vi "Gestione_Inverter_VACON.vi"(6 "Inverter":refnum<vi>, 7 "Stato rpm":refnum<vi>, 8 "Test settings":refnum<vi>, 9 "RS485":refnum<vi>, 11 "name":string="VACON") -> ()   [LabVIEW 2019]
uses:
  Letture inverter.ctl
  Parametri inverter.ctl
  <vilib>/Modbus/subvis/Modbus API/Modbus API.lvclass/Modbus API.ctl
  <vilib>/Modbus/subvis/Transmission Data Unit (ADU)/Transmission Data Unit/Transmission Data Unit.lvclass/Transmission Data Unit.ctl
  <vilib>/Modbus/master/Data Access/Unit ID/Set Unit ID Property.vi
  <vilib>/Modbus/subvis/Transmission Data Unit (ADU)/Transmission Data Unit/Data Access/Unit ID/Write Unit ID.vi
  <vilib>/Modbus/subvis/Modbus API/Read Transmission Data Unit.vi
  <vilib>/Modbus/subvis/Modbus API/Write Transmission Data Unit.vi
  <vilib>/Modbus/master/Modbus Master.lvclass
  C:/Program Files (x86)/National Instruments/LabVIEW 2019/vi.lib/Modbus/subvis/Modbus API/Modbus API.lvclass
  <vilib>/Utility/file.llb/Read From Spreadsheet File (string).vi
  <vilib>/Modbus/master/Create Master Instance (Serial).vi
  STATUS VACON.vi
  <vilib>/Modbus/subvis/Transmission Data Unit (ADU)/Transmission Data Unit/Transmission Data Unit.lvclass
  Set inverter.ctl
panel:
  out "Cluster":T1
  out "senso rot":bool
  out "Boolean array":bool[](array[boolean])
  out "STATUS WORD":u16
  out "fREQ MAX":dbl
  in  "SET INVERTER":bool
  in  "Test settings 2":T2 caption="PARAMETRI INVERTER"
  in  "Scelta inverter":T3(radio)=enum."INVERTER 1 \n[7,5kW]"
  out "id":u8
  in  "stop":bool
  out "Numeric":i32
  out "status":string
  out "output cluster":T4
  out "error out":errorcluster
  # "Caratteristiche motore"
  # "Limiti massimi"
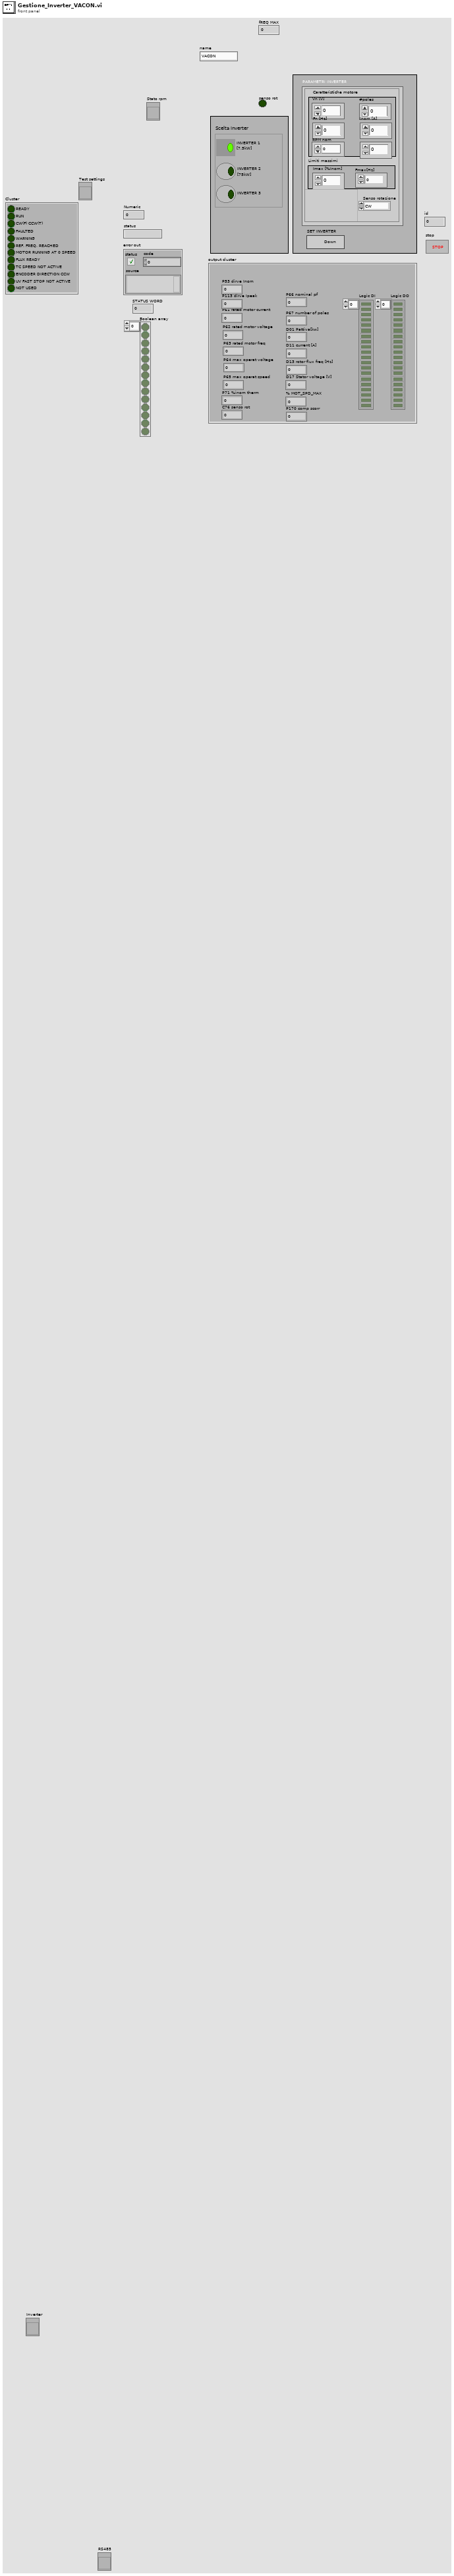
[diagram p1: front panel]
types:
  T1 = cluster{"READY":bool, "RUN":bool, "CW(F) CCW(T)":bool, "FAULTED":bool, "WARNING":bool, "REF. FREQ. REACHED":bool, "MOTOR RUNNING AT 0 SPEED":bool, "FLUX READY":bool, "TC SPEED NOT ACTIVE":bool, "ENCODER DIRECTION CCW":bool, "UV FAST STOP NOT ACTIVE":bool, "NOT USED":bool}
  T2 = typedef "Parametri inverter.ctl" = cluster{"Vn [V]":dbl, "Fn [Hz]":dbl, "CosFi":dbl, "Imax [%Inom]":dbl, "#poles":dbl, "Inom [A]":dbl, "Senso rotazione":enum16{"CW", "CCW"}, "RPM nom":dbl, "Fmax[Hz]":dbl}
  T3 = enum32{"No Selection", "INVERTER 1 \n[7,5kW]", "INVERTER 2 \n[75kW]", "INVERTER 3"}
  T4 = typedef "Letture inverter.ctl" = cluster{"P61 rated motor current":dbl, "P62 rated motor voltage":dbl, "P63 rated motor freq":dbl, "P64 max operat voltage":dbl, "P65 max operat speed":dbl, "P66 nominal pf":dbl, "P67 number of poles":dbl, "D01 Pattiva[kw]":dbl, "D11 current [A]":dbl, "D13 rotor flux freq [Hz]":dbl, "D17 Stator voltage [V]":dbl, "% MOT_SPD_MAX":dbl, "Logic DI":bool[], "Logic DO":bool[], "P71 %inom therm":dbl, "P53 dirve Inom":dbl, "P113 dirve Ipeak":dbl, "C76 senso rot":dbl, "P170 comp scorr":dbl}
  T5 = typedef "Set inverter.ctl" = cluster{"F [Hz]":dbl}
  T6 = cluster{"Boolean array[0]":bool, "Boolean array[1]":bool, "Boolean array[2]":bool, "Boolean array[3]":bool, "Boolean array[4]":bool, "Boolean array[5]":bool, "Boolean array[6]":bool, "Boolean array[7]":bool, "Boolean array[8]":bool, "Boolean array[9]":bool, "Boolean array[10]":bool, "Boolean array[11]":bool}
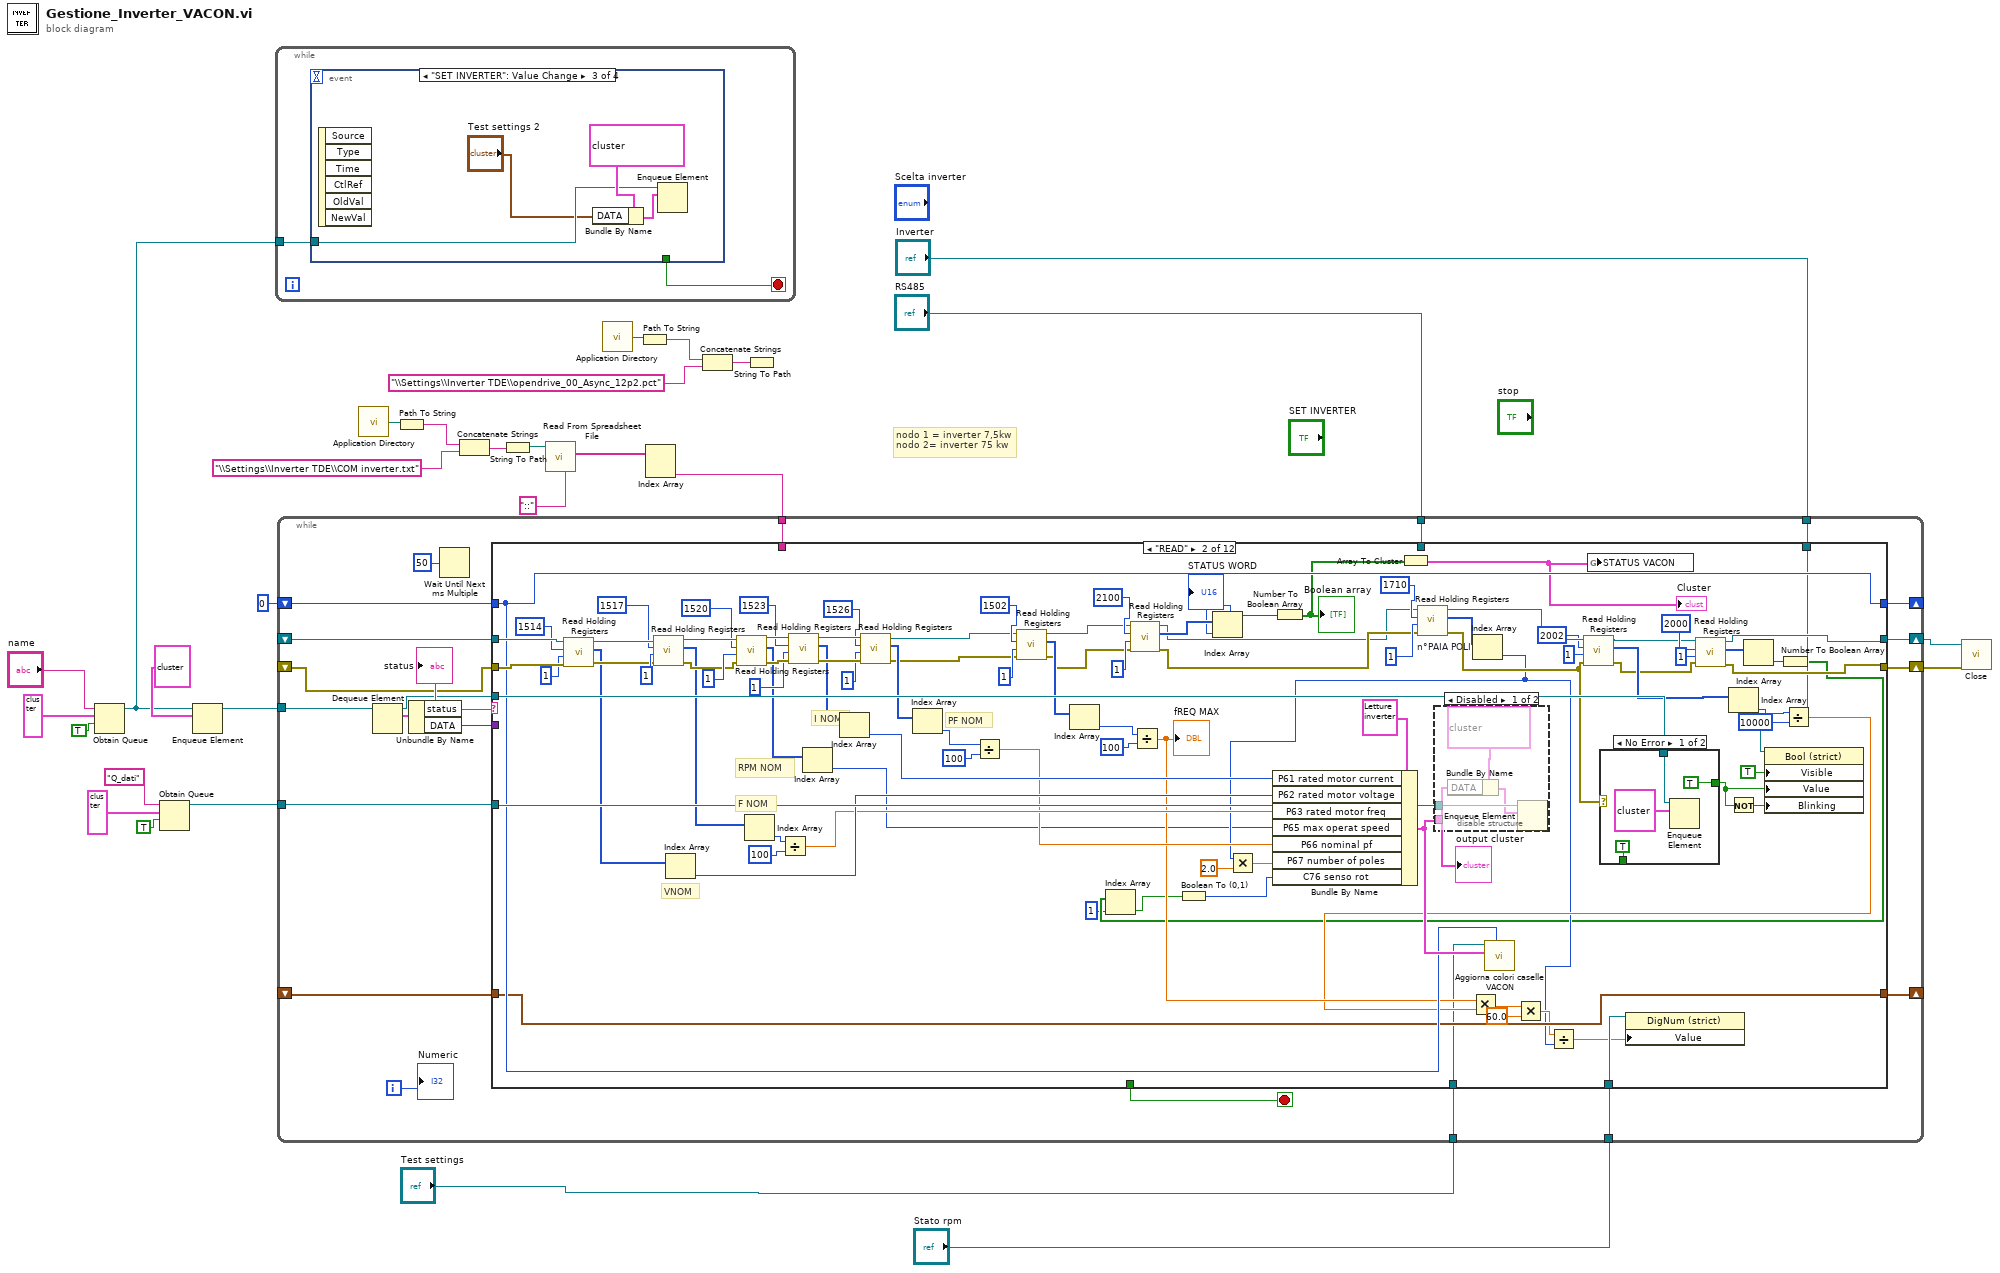
[diagram p0: block diagram]
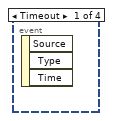
[diagram p2: hidden frame]
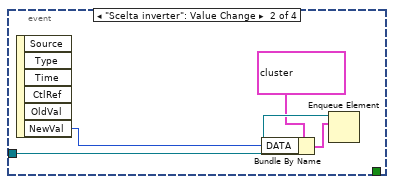
[diagram p3: hidden frame]
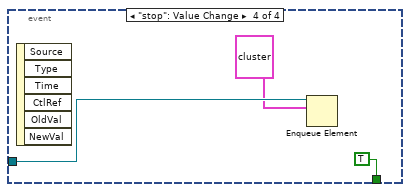
[diagram p4: hidden frame]
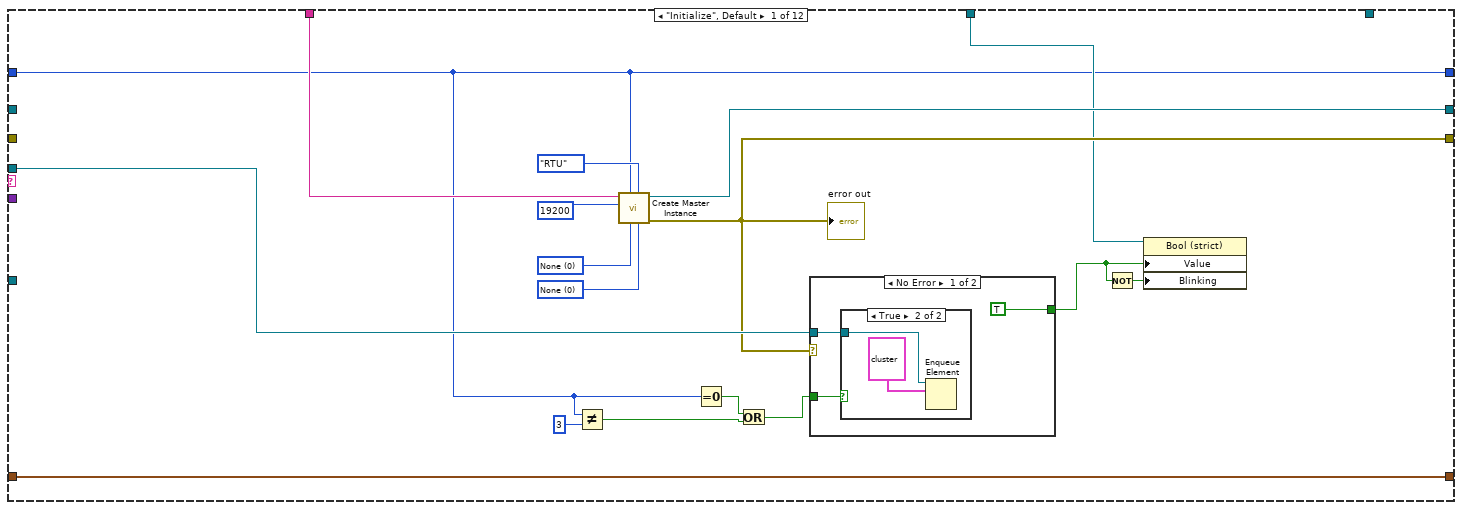
[diagram p5: hidden frame]
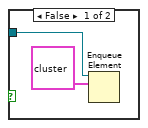
[diagram p6: hidden frame]
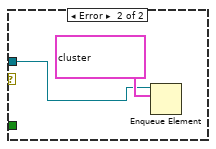
[diagram p7: hidden frame]
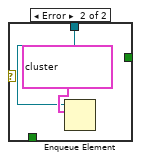
[diagram p9: hidden frame]
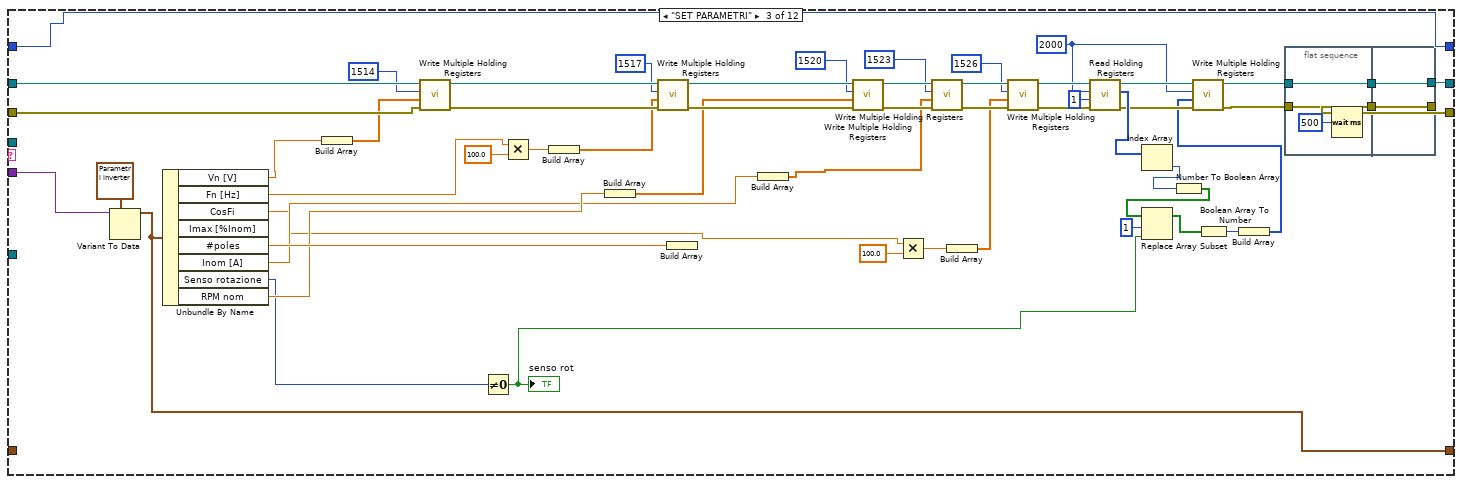
[diagram p10: hidden frame]
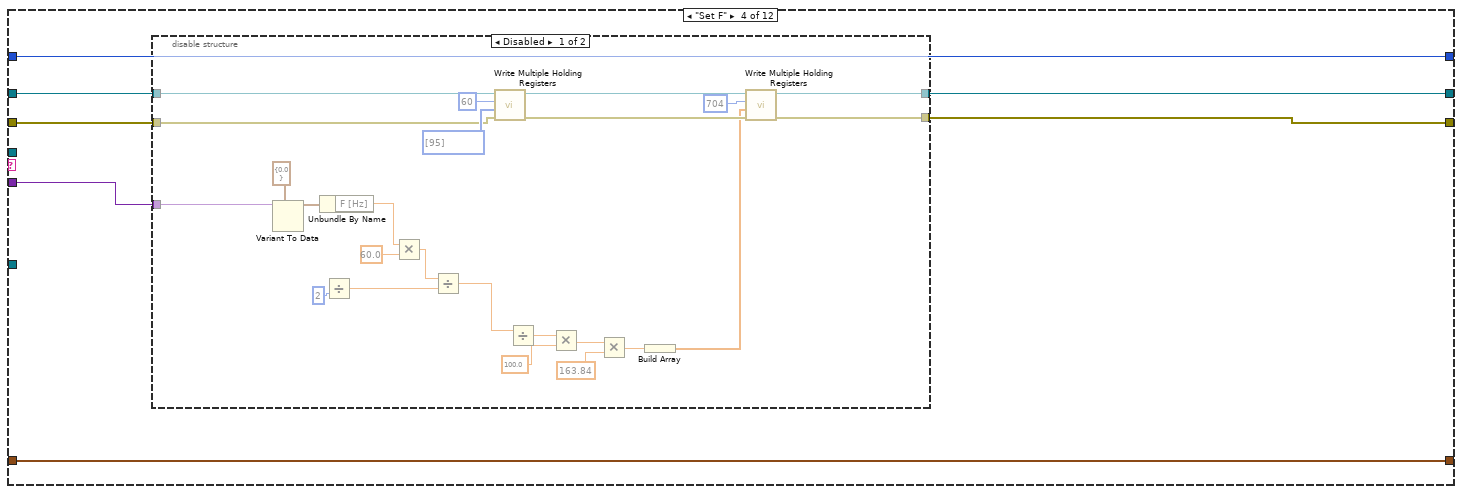
[diagram p11: hidden frame]
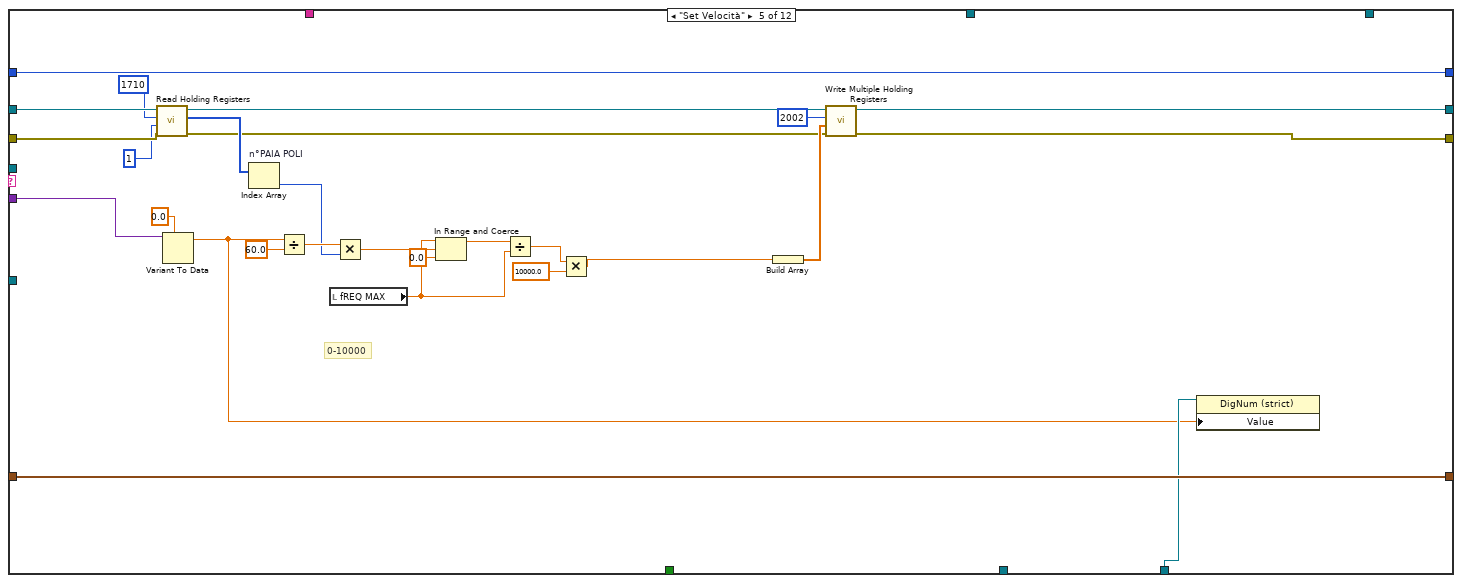
[diagram p13: hidden frame]
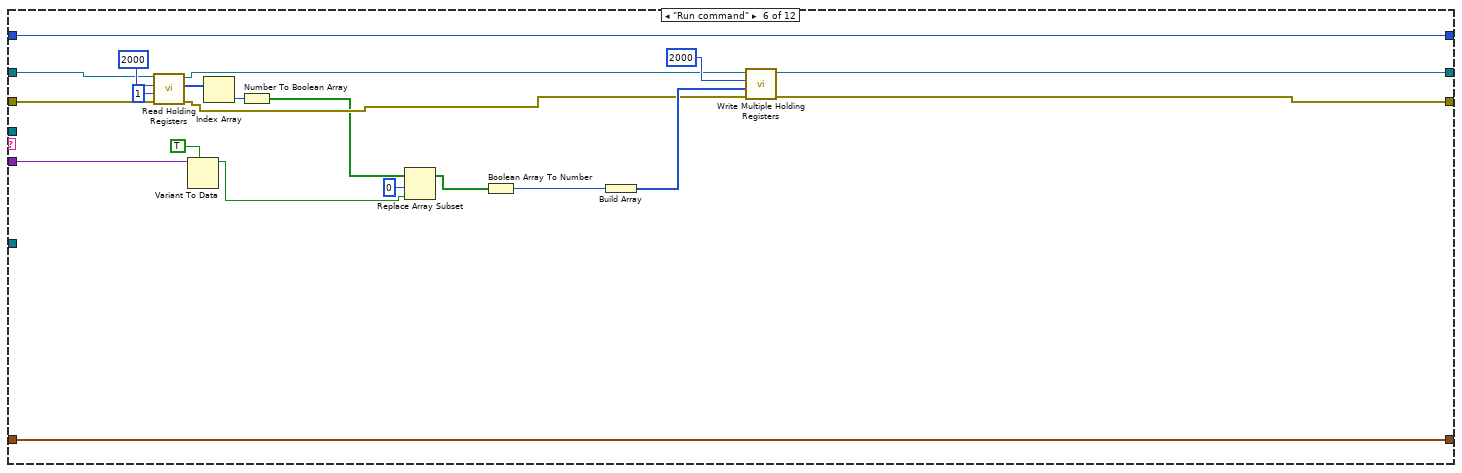
[diagram p14: hidden frame]
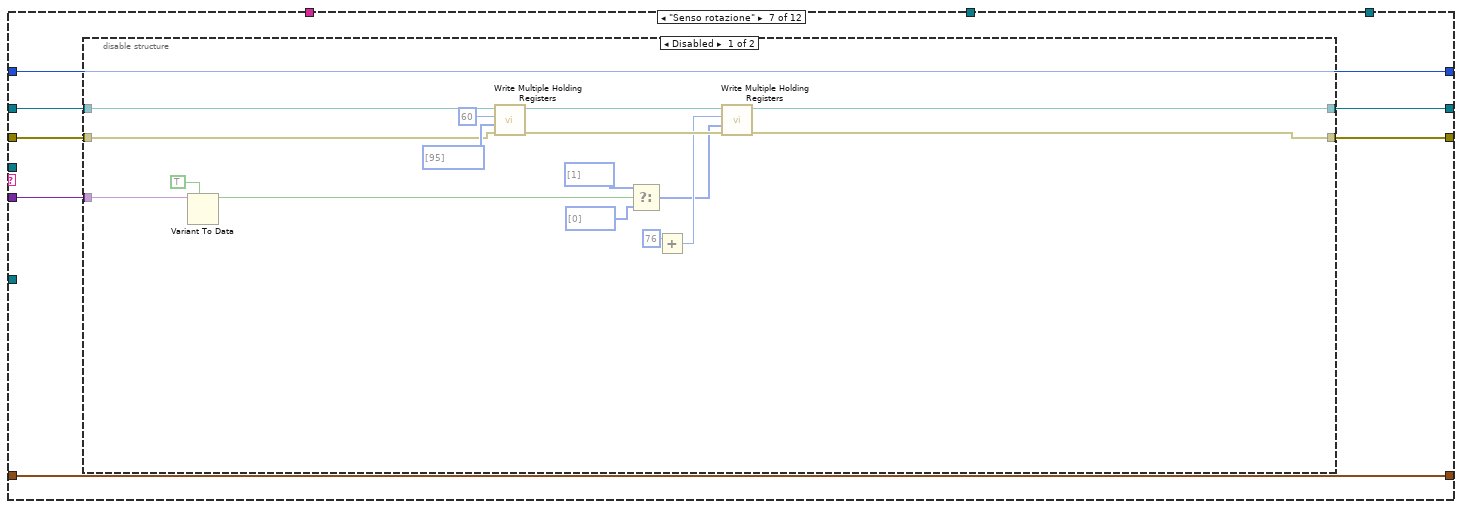
[diagram p15: hidden frame]
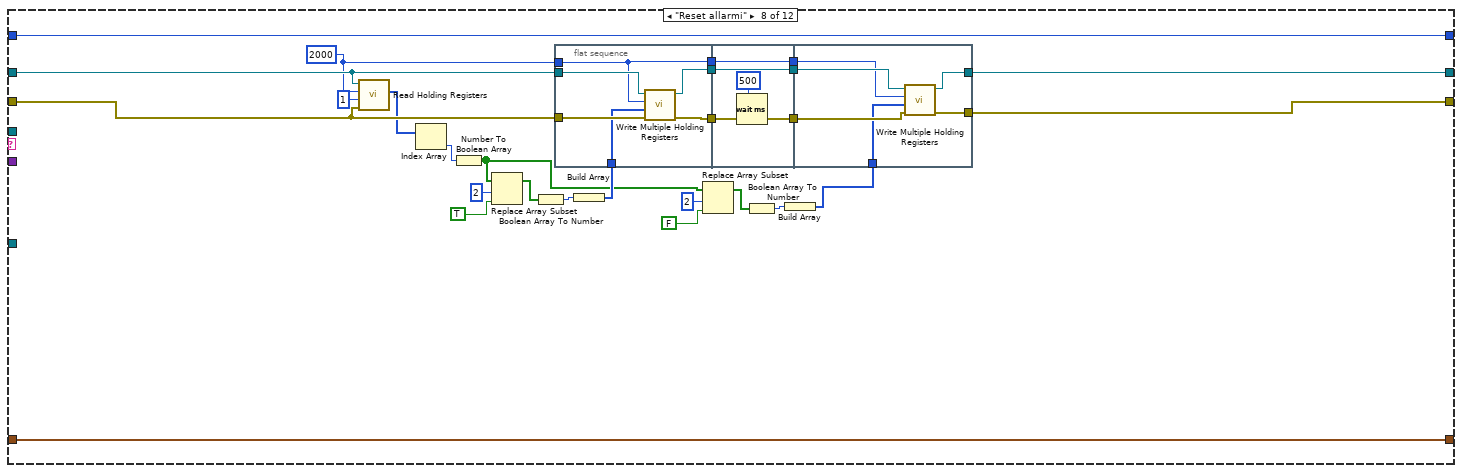
[diagram p17: hidden frame]
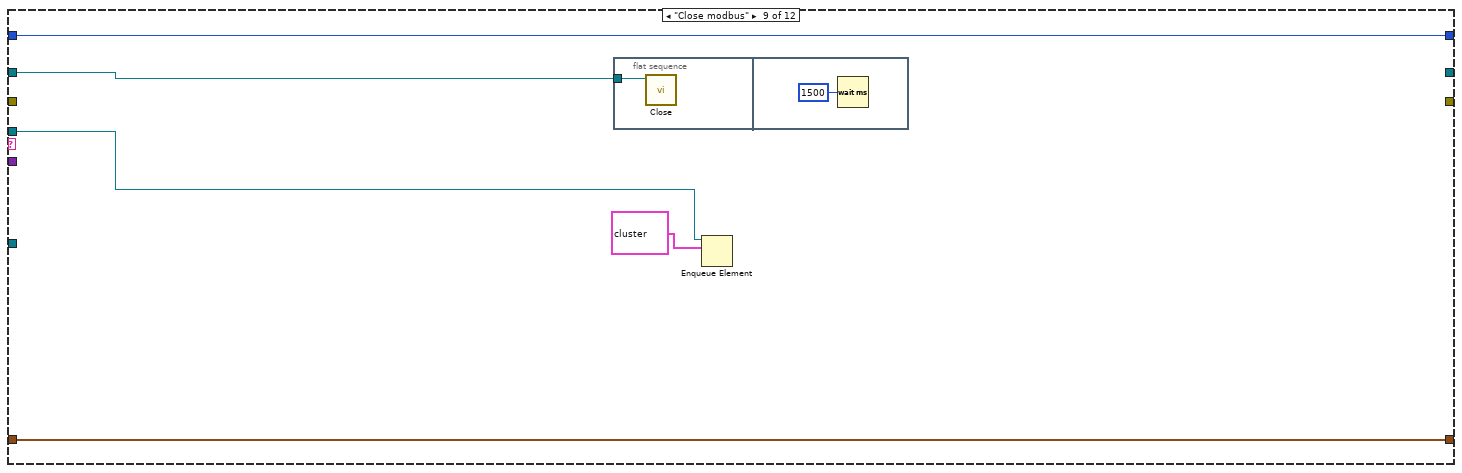
[diagram p18: hidden frame]
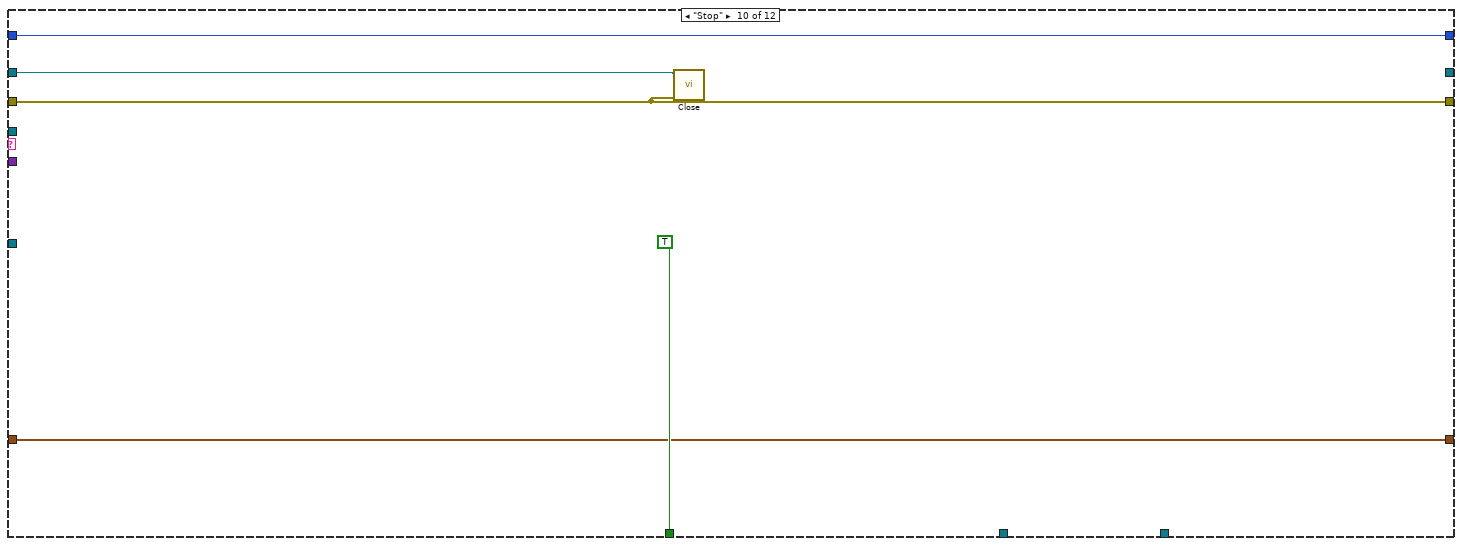
[diagram p19: hidden frame]
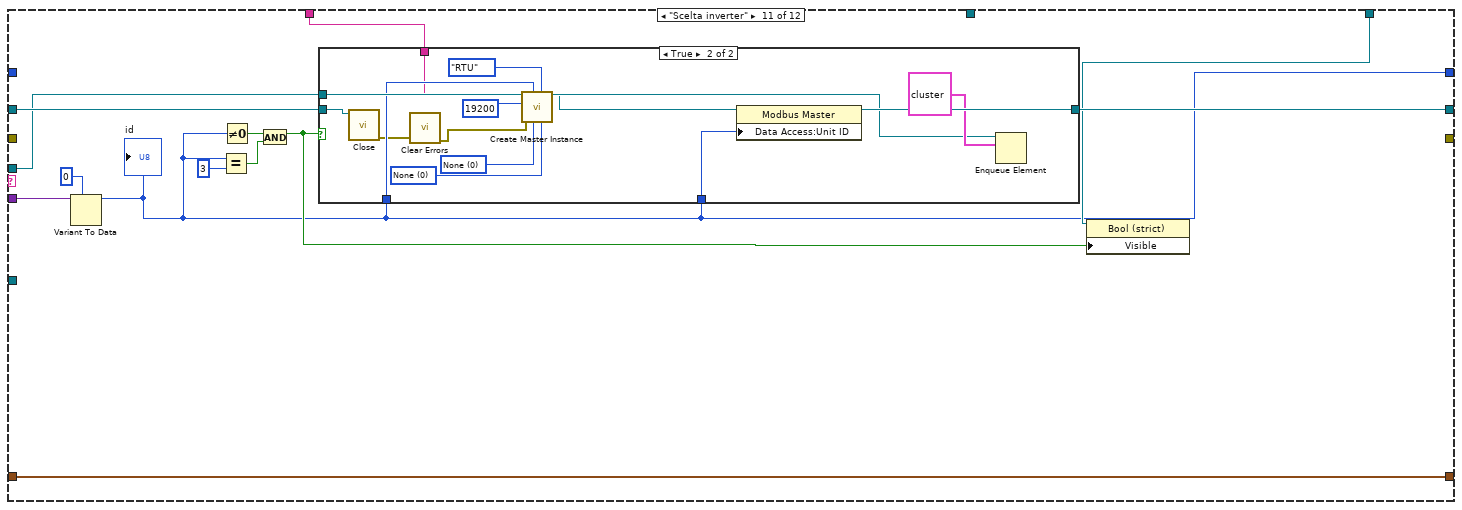
[diagram p20: hidden frame]
diagram:
  # "nodo 1 = inverter 7,5kw\nnodo 2= inverter 75 kw"
  n1 = Obtain Queue(name (unnamed)="name", element data type=cluster{"DATA":variant, "status":string} {"DATA"=variant, "status"=""} ("output cluster"), create if not found? (T)=TRUE) -> (queue out=w5:refnum<queue>)  [unwired: 2 in, 2 out]
  n2 = Obtain Queue(name (unnamed)="Q_dati", element data type=cluster{"DATA":variant, "status":string} {"DATA"=variant, "status"=""} ("output cluster"), create if not found? (T)=TRUE) -> (queue out=w23:refnum<queue>)  [unwired: 2 in, 2 out]
  n3 = Enqueue Element(queue=w5, element=cluster{"DATA":variant, "status":string} {"DATA"=variant, "status"="IDLE"}) -> (queue out=w21:refnum<queue>)  [unwired: 2 in, 2 out]
  n4 = while {
    tunnel: w5 -> [w31]
    stop <- w30 stop-if-true
    n5 = event shown="[2] \"SET INVERTER\": Value Change" {
      selector: _ -> [_ _ _ _]
      dyn-events: _ -> [_ _ _ _]
      timeout: _ -> [_ _ _ _]
      tunnel: w31 -> [_ w35 w37 w42]
      tunnel: [_ _ _ TRUE] -> w30
      event Timeout {
        n6 = event-data() -> ()  [unwired: 1 in, 3 out]
      }
      event "Scelta inverter": Value Change {
        n7 = event-data() -> ("NewVal"=w32:T3)  [unwired: 1 in, 5 out]
        n8 = Bundle By Name(cluster=cluster{"DATA":variant, "status":string} {"DATA"=variant, "status"="Scelta inverter"} ("element"), "DATA"=w32) -> (w33:cluster{"DATA":variant, "status":string})
        n9 = Enqueue Element(queue=w35, element=w33) -> ()  [unwired: 2 in, 3 out]
      }
      event "SET INVERTER": Value Change {
        n10 = event-data() -> ()  [unwired: 1 in, 6 out]
        n11 = Bundle By Name(cluster=cluster{"DATA":variant, "status":string} {"DATA"=variant, "status"="SET PARAMETRI"} ("element"), "DATA"="Test settings 2") -> (w38:cluster{"DATA":variant, "status":string})
        n12 = Enqueue Element(queue=w37, element=w38) -> ()  [unwired: 2 in, 3 out]
      }
      event "stop": Value Change {
        n13 = event-data() -> ()  [unwired: 1 in, 6 out]
        n14 = Enqueue Element(queue=w42, element=cluster{"DATA":variant, "status":string} {"DATA"=variant, "status"="Stop"}) -> ()  [unwired: 2 in, 3 out]
      }
    }
  }
  n15 = call <vilib>:"Application Directory.vi"() -> ("Application Directory"=w13:path)
  n16 = Path To String(path=w13) -> (string=w14:string)
  n17 = Concatenate Strings(w14, "\\Settings\\Inverter TDE\\COM inverter.txt" ("name or relative path")) -> (w16:string)
  n18 = String To Path(string=w16) -> (path=w17:path)
  n19 = call-poly <vilib>:"Read From Spreadsheet File.vi"("delimiter (\\t)"="::" ("delimiter (\\t)"), "file path (dialog if empty)"=w17) -> ("first row"=w11:string[])  [unwired: 5 in, 4 out]
  n20 = call <vilib>:"Application Directory.vi"() -> ("Application Directory"=w9:path)
  n21 = Path To String(path=w9) -> (string=w8:string)
  n22 = Index Array(array=w11) -> (element #2=w10:string)  [unwired: 2 in, 1 out]
  n23 = while {
    tunnel: w21 -> [w64]
    shift-right: [w59] -> w19
    shift-left: _ -> [w45]
    shift-right: [w58] -> w20
    shift-left: _ -> [w49]
    tunnel: w23 -> [w57]
    tunnel: "RS485" -> [w53]
    tunnel: w10 -> [w52]
    shift-right: [w51] -> _
    shift-left: _ -> [w50]
    tunnel: "Test settings" -> [w48]
    shift-right: [w47] -> _
    shift-left: u8 0 ("unit ID") -> [w46]
    tunnel: "Inverter" -> [w44]
    tunnel: "Stato rpm" -> [w43]
    i -> [w54]
    stop <- w60 stop-if-true
    n24 = Dequeue Element(queue=w64) -> (queue out=w55:refnum<queue>, element=w63:cluster{"DATA":variant, "status":string})  [unwired: 2 in, 2 out]
    n25 = Unbundle By Name(w63) -> ("status"=w62:string, "DATA"=w61:variant)
    "status" <- w62
    n26 = Wait Until Next ms Multiple(millisecond multiple=u32 50) -> ()  [unwired: 1 out]
    n27 = case shown="\"READ\"" w62 {
      tunnel: w61 -> [_ _ w249 w257 w310 w331 w336 _ _ _ w421 _]
      tunnel: [_ _ _ _ _ _ _ _ _ TRUE _ _] -> w60
      tunnel: [w81 w97 w246 w259 w312 w333 w338 w383 _ _ w422 w444] -> w59
      tunnel: [w75 w96 w245 w258 w311 w332 w337 w382 _ w409 _ w443] -> w58
      tunnel: w45 -> [_ w172 w248 w261 w307 w316 w340 w375 w404 w410 w423 w444]
      tunnel: w49 -> [_ w174 w247 w260 w306 w317 w339 w374 _ w409 _ w443]
      tunnel: w57 -> [_ w184 _ _ _ _ _ _ _ _ _ _]
      tunnel: w55 -> [w76 w181 _ _ _ _ _ _ w402 _ w419 _]
      tunnel: w53 -> [w73 _ _ _ _ _ _ _ _ _ _ _]
      tunnel: w52 -> [w70 _ _ _ _ _ _ _ _ _ w412 _]
      tunnel: [w71 w167 w244 w256 w309 w330 w335 w381 w401 w408 w424 w446] -> w51
      tunnel: w50 -> [w71 w167 _ w256 w309 w330 w335 w381 w401 w408 w424 w446]
      tunnel: w46 -> [w68 w168 w243 w255 w308 w322 w334 w380 w400 w407 _ w445]
      tunnel: w48 -> [_ w91 _ _ _ _ _ _ _ _ _ _]
      tunnel: [w68 w168 w243 w255 w308 w322 w334 w380 w400 w407 w413 w445] -> w47
      tunnel: w44 -> [_ w95 _ _ _ _ _ _ _ _ w418 _]
      tunnel: w43 -> [_ w163 _ _ w291 _ _ _ _ _ _ _]
      frame "Initialize", Default {
        w78 = u16 0 items=["None", "XON/XOFF", "RTS/CTS", "XON/XOFF & RTS/CTS", "DTR/DSR", "XON/XOFF & DTR/DSR"] ("flow control (None)")
        w79 = u16 0 items=["None", "Odd", "Even"] ("parity (Even)")
        n28 = Not Equal?(x=w68, y=u8 3) -> (x != y?=w66:bool)
        n29 = call-poly <vilib>:"Create Master Instance.vi"("flow control (None)"=w78, "serial type"=enum16{"RTU", "ASCII"}."RTU", "parity (Even)"=w79, "unit ID"=w68, "baud rate (9600)"=u32 19200, "VISA resource name"=w70) -> ("error out"=w75:errorcluster, "serial master instance"=w81:refnum<class "Modbus Master.lvclass">)  [unwired: 4 in]
        "error out" <- w75
        n30 = Equal To 0?(x=w68) -> (x = 0?=w69:bool)
        n31 = Or(x=w69, y=w66) -> (x .or. y?=w65:bool)
        n32 = case shown="No Error" w75 {
          tunnel: w76 -> [w84 w89]
          tunnel: [TRUE _] -> w72
          tunnel: w65 -> [w82 _]
          frame No Error {
            n33 = case shown="True" w82 {
              tunnel: w84 -> [w85 w88]
              frame False {
                n34 = Enqueue Element(queue=w85, element=cluster{"DATA":variant, "status":string} {"DATA"=variant, "status"="READ"}) -> ()  [unwired: 2 in, 3 out]
              }
              frame True {
                n35 = Enqueue Element(queue=w88, element=cluster{"DATA":variant, "status":string} {"DATA"=variant, "status"="IDLE"}) -> ()  [unwired: 2 in, 3 out]
              }
            }
          }
          frame Error {
            n36 = Enqueue Element(queue=w89, element=cluster{"DATA":variant, "status":string} {"DATA"=variant, "status"="Close modbus"}) -> ()  [unwired: 2 in, 3 out]
          }
        }
        n37 = Not(x=w72) -> (.not. x?=w74:bool)
        n38 = property class="Bool (strict)"(reference=w73, "Value"=w72, "Blinking"=w74) -> ()  [unwired: 1 in, 2 out]
      }
      frame "READ" {
        # "PF NOM"
        # "I NOM"
        # "RPM NOM"
        # "F NOM"
        # "VNOM"
        n39 = call-dynamic "Read Holding Registers.vi"("error in (no error)"=w174, "number of holding registers"=u16 1, "starting address"=1514 ("x"), "Modbus master in"=w172) -> ("error out"=w173:errorcluster, "register values"=w170:u16[], "Modbus master out"=w171:refnum<class "Modbus Master.lvclass">)  [unwired: 5 in]
        n40 = call-dynamic "Read Holding Registers.vi"("error in (no error)"=w173, "number of holding registers"=u16 1, "starting address"=1517 ("x"), "Modbus master in"=w171) -> ("error out"=w179:errorcluster, "register values"=w177:u16[], "Modbus master out"=w180:refnum<class "Modbus Master.lvclass">)  [unwired: 5 in]
        n41 = Index Array(array=w170) -> (element=w155:u16)  [unwired: 1 in]
        n42 = call-dynamic "Read Holding Registers.vi"("error in (no error)"=w179, "number of holding registers"=u16 1, "starting address"=u16 1520, "Modbus master in"=w180) -> ("error out"=w160:errorcluster, "register values"=w151:u16[], "Modbus master out"=w162:refnum<class "Modbus Master.lvclass">)  [unwired: 5 in]
        n43 = Index Array(array=w177) -> (element=w176:u16)  [unwired: 1 in]
        n44 = Divide(x=w176, y=u16 100) -> (x/y=w153:dbl)
        n45 = call-dynamic "Read Holding Registers.vi"("error in (no error)"=w160, "number of holding registers"=u16 1, "starting address"=u16 1523, "Modbus master in"=w162) -> ("error out"=w159:errorcluster, "register values"=w149:u16[], "Modbus master out"=w161:refnum<class "Modbus Master.lvclass">)  [unwired: 5 in]
        n46 = Index Array(array=w151) -> (element=w106:u16)  [unwired: 1 in]
        n47 = Index Array(array=w149) -> (element=w148:u16)  [unwired: 1 in]
        n48 = call-dynamic "Read Holding Registers.vi"("error in (no error)"=w159, "number of holding registers"=u16 1, "starting address"=u16 1526, "Modbus master in"=w161) -> ("error out"=w137:errorcluster, "register values"=w145:u16[], "Modbus master out"=w138:refnum<class "Modbus Master.lvclass">)  [unwired: 5 in]
        n49 = Index Array(array=w145) -> (element=w143:u16)  [unwired: 1 in]
        n50 = Divide(x=w143, y=u16 100) -> (x/y=w142:dbl)
        n51 = call-dynamic "Read Holding Registers.vi"("error in (no error)"=w137, "number of holding registers"=u16 1, "starting address"=u16 1502, "Modbus master in"=w138) -> ("error out"=w131:errorcluster, "register values"=w141:u16[], "Modbus master out"=w132:refnum<class "Modbus Master.lvclass">)  [unwired: 5 in]
        n52 = Index Array(array=w141) -> (element=w135:u16)  [unwired: 1 in]
        n53 = call-dynamic "Read Holding Registers.vi"("error in (no error)"=w131, "number of holding registers"=u16 1, "starting address"=u16 2100, "Modbus master in"=w132) -> ("error out"=w125:errorcluster, "register values"=w130:u16[], "Modbus master out"=w124:refnum<class "Modbus Master.lvclass">)  [unwired: 5 in]
        n54 = Divide(x=w135, y=u16 100) -> (x/y=w113:dbl)
        "fREQ MAX" <- w113
        n55 = Index Array(array=w130) -> (element=w129:u16)  [unwired: 1 in]
        "STATUS WORD" <- w129
        n56 = Number To Boolean Array(number=w129) -> (Boolean array=w121:bool[])
        "Boolean array" <- w121
        n57 = Array To Cluster(array=w121) -> (cluster=w105:T6)
        "Cluster" <- w105
        n58 = call-dynamic "Read Holding Registers.vi"("error in (no error)"=w125, "number of holding registers"=u16 1, "starting address"=u16 1710, "Modbus master in"=w124) -> ("error out"=w119:errorcluster, "register values"=w127:u16[], "Modbus master out"=w120:refnum<class "Modbus Master.lvclass">)  [unwired: 5 in]
        n59 = Index Array "n°PAIA POLI"(array=w127) -> (element=w108:u16)  [unwired: 1 in]
        n60 = Multiply(x=w108, y=2.0) -> (x*y=w123:dbl)
        n61 = call-dynamic "Read Holding Registers.vi"("error in (no error)"=w119, "number of holding registers"=u16 1, "starting address"=u16 2002, "Modbus master in"=w120) -> ("error out"=w98:errorcluster, "register values"=w116:u16[], "Modbus master out"=w99:refnum<class "Modbus Master.lvclass">)  [unwired: 5 in]
        n62 = global write "STATUS VACON.vi" "STATUS VACON"(w105) -> ()
        n63 = case shown="No Error" w119 {
          tunnel: w181 -> [w191 w193]
          tunnel: [TRUE _] -> _
          tunnel: [TRUE _] -> w165
          frame No Error {
            n64 = Enqueue Element(queue=w191, element=cluster{"DATA":variant, "status":string} {"DATA"=variant, "status"="READ"}) -> ()  [unwired: 2 in, 3 out]
          }
          frame Error {
            n65 = Enqueue Element(queue=w193, element=cluster{"DATA":variant, "status":string} {"DATA"=variant, "status"="Close modbus"}) -> ()  [unwired: 2 in, 3 out]
          }
        }
        n66 = call-dynamic "Read Holding Registers.vi"("error in (no error)"=w98, "number of holding registers"=u16 1, "starting address"=u16 2000, "Modbus master in"=w99) -> ("error out"=w96:errorcluster, "register values"=w102:u16[], "Modbus master out"=w97:refnum<class "Modbus Master.lvclass">)  [unwired: 5 in]
        n67 = Index Array(array=w116) -> (element=w115:u16)  [unwired: 1 in]
        n68 = Not(x=w165) -> (.not. x?=w166:bool)
        n69 = Index Array(array=w102) -> (element=w101:u16)  [unwired: 1 in]
        n70 = property class="Bool (strict)"(reference=w95, "Visible"=TRUE, "Value"=w165, "Blinking"=w166) -> ()  [unwired: 1 in, 2 out]
        n71 = Number To Boolean Array(number=w101) -> (Boolean array=w94:bool[])
        n72 = Index Array(array=w94, index=1) -> (element=w92:bool)
        n73 = Boolean To (0,1)(Boolean=w92) -> (0, 1=w104:i16)
        n74 = Bundle By Name(cluster=T4 {"P61 rated motor current"=0.0, "P62 rated motor voltage"=0.0, "P63 rated motor freq"=0.0, "P64 max operat voltage"=0.0, "P65 max operat speed"=0.0, "P66 nominal pf"=0.0, "P67 number of poles"=0.0, "D01 Pattiva[kw]"=0.0, "D11 current [A]"=0.0, "D13 rotor flux freq [Hz]"=0.0, "D17 Stator voltage [V]"=0.0, "% MOT_SPD_MAX"=0.0, "Logic DI"=[], "Logic DO"=[], "P71 %inom therm"=0.0, "P53 dirve Inom"=0.0, "P113 dirve Ipeak"=0.0, "C76 senso rot"=0.0, "P170 comp scorr"=0.0} ("Letture inverter"), "P61 rated motor current"=w148, "P62 rated motor voltage"=w155, "P63 rated motor freq"=w153, "P65 max operat speed"=w106, "P66 nominal pf"=w142, "P67 number of poles"=w123, "C76 senso rot"=w104) -> (w169:T4)
        "output cluster" <- w169
        n75 = disable-structure shown="Disabled" {
          disable-tunnel: w184 -> [w188 _]
          disable-tunnel: w169 -> [w185 _]
          frame Disabled {
            n76 = Bundle By Name(cluster=cluster{"DATA":variant, "status":string} {"DATA"=variant, "status"="Leggi inverter"} ("element"), "DATA"=w185) -> (w187:cluster{"DATA":variant, "status":string})
            n77 = Enqueue Element(queue=w188, element=w187) -> ()  [unwired: 2 in, 3 out]
          }
          frame Enabled {
          }
        }
        n78 = call "Aggiorna colori caselle VACON.vi"("id"=w168, "Letture inverter"=w169, "Test settings"=w91) -> ()  [unwired: 9 in]
        n79 = Divide(x=w115, y=u16 10000) -> (x/y=w112:dbl)
        n80 = Multiply(x=w113, y=w112) -> (x*y=w111:dbl)
        n81 = Multiply(x=w111, y=60.0) -> (x*y=w109:dbl)
        n82 = Divide(x=w109, y=w108) -> (x/y=w107:dbl)
        n83 = property class="DigNum (strict)"(reference=w163, "Value"=w107) -> ()  [unwired: 1 in, 2 out]
      }
      frame "SET PARAMETRI" {
        w197 = u16 2000 ("starting address")
        n84 = Variant To Data(type=T2 {"Vn [V]"=400.0, "Fn [Hz]"=50.0, "CosFi"=65.0, "Imax [%Inom]"=65.0, "#poles"=4.0, "Inom [A]"=0.0, "Senso rotazione"=enum."CW", "RPM nom"=0.0, "Fmax[Hz]"=0.0} ("Test settings"), Variant=w249) -> (data=w244:T2)  [unwired: 1 in, 1 out]
        n85 = Unbundle By Name(w244) -> ("Vn [V]"=w223:dbl, "Fn [Hz]"=w222:dbl, "CosFi"=w211:dbl, "#poles"=w229:dbl, "Inom [A]"=w217:dbl, "Senso rotazione"=w212:enum16{"CW", "CCW"}, "RPM nom"=w220:dbl)  [unwired: 1 out]
        n86 = Build Array(w223) -> (w228:dbl[])
        n87 = call-dynamic "Write Multiple Holding Registers.vi"("error in (no error)"=w247, "holding register values"=w228, "starting address"=u16 1514 ("write operation starting address"), "Modbus master in"=w248) -> ("error out"=w238:errorcluster, "Modbus master out"=w237:refnum<class "Modbus Master.lvclass">)  [unwired: 6 in]
        n88 = Not Equal To 0?(x=w212) -> (x != 0?=w203:bool)
        "senso rot" <- w203
        n89 = Multiply(x=w222, y=100.0) -> (x*y=w225:dbl)
        n90 = Build Array(w225) -> (w224:dbl[])
        n91 = Build Array(w220) -> (w219:dbl[])
        n92 = call-dynamic "Write Multiple Holding Registers.vi"("error in (no error)"=w238, "holding register values"=w224, "starting address"=1517 ("x"), "Modbus master in"=w237) -> ("error out"=w236:errorcluster, "Modbus master out"=w235:refnum<class "Modbus Master.lvclass">)  [unwired: 6 in]
        n93 = Build Array(w229) -> ()  [unwired: 1 out]
        n94 = Build Array(w217) -> (w216:dbl[])
        n95 = call-dynamic "Write Multiple Holding Registers.vi"("error in (no error)"=w236, "holding register values"=w219, "starting address"=1520 ("x"), "Modbus master in"=w235) -> ("error out"=w233:errorcluster, "Modbus master out"=w234:refnum<class "Modbus Master.lvclass">)  [unwired: 6 in]
        n96 = Multiply(x=w211, y=100.0) -> (x*y=w213:dbl)
        n97 = call-dynamic "Write Multiple Holding Registers.vi"("error in (no error)"=w233, "holding register values"=w216, "starting address"=1523 ("x"), "Modbus master in"=w234) -> ("error out"=w232:errorcluster, "Modbus master out"=w231:refnum<class "Modbus Master.lvclass">)  [unwired: 6 in]
        n98 = Build Array(w213) -> (w230:dbl[])
        n99 = call-dynamic "Write Multiple Holding Registers.vi"("error in (no error)"=w232, "holding register values"=w230, "starting address"=1526 ("x"), "Modbus master in"=w231) -> ("error out"=w209:errorcluster, "Modbus master out"=w210:refnum<class "Modbus Master.lvclass">)  [unwired: 6 in]
        n100 = call-dynamic "Read Holding Registers.vi"("error in (no error)"=w209, "number of holding registers"=u16 1, "starting address"=w197, "Modbus master in"=w210) -> ("error out"=w201:errorcluster, "register values"=w207:u16[], "Modbus master out"=w199:refnum<class "Modbus Master.lvclass">)  [unwired: 5 in]
        n101 = Index Array(array=w207) -> (element=w206:u16)  [unwired: 1 in]
        n102 = Number To Boolean Array(number=w206) -> (Boolean array=w205:bool[])
        n103 = Replace Array Subset(array=w205, new element=w203, index=1) -> (w202:bool[])
        n104 = Boolean Array To Number(Boolean array=w202) -> (number=w196:u32)
        n105 = Build Array(w196) -> (w195:u32[])
        n106 = call-dynamic "Write Multiple Holding Registers.vi"("error in (no error)"=w201, "holding register values"=w195, "starting address"=w197, "Modbus master in"=w199) -> ("error out"=w200:errorcluster, "Modbus master out"=w198:refnum<class "Modbus Master.lvclass">)  [unwired: 6 in]
        n107 = flat-sequence {
          tunnel: w200 -> [w251]
          tunnel: w198 -> [w252]
          tunnel: [w252] -> w242
          tunnel: [w251] -> w241
          tunnel: [w254] -> w246
          tunnel: [w253] -> w245
          tunnel: w242 -> [w254]
          tunnel: w241 -> [w253]
          frame #0 {
            n108 = Wait (ms)(milliseconds to wait=u32 500) -> ()  [unwired: 1 out]
          }
          frame #1 {
          }
        }
      }
      frame "Set F" {
        n109 = disable-structure shown="Disabled" {
          disable-tunnel: w261 -> [w280 _]
          disable-tunnel: w260 -> [w279 _]
          disable-tunnel: [w278 _] -> w259
          disable-tunnel: [w277 _] -> w258
          disable-tunnel: w257 -> [w276 _]
          frame Disabled {
            n110 = Variant To Data(type=T5 {"F [Hz]"=0.0} ("Set inverter"), Variant=w276) -> (data=w274:T5)  [unwired: 1 in, 1 out]
            n111 = Unbundle By Name(w274) -> ("F [Hz]"=w273:dbl)
            n112 = Divide(y=u16 2) -> (x/y=w269:dbl)  [unwired: 1 in]
            n113 = Multiply(x=w273, y=60.0) -> (x*y=w271:dbl)
            n114 = Divide(x=w271, y=w269) -> (x/y=w262:dbl)
            n115 = call-dynamic "Write Multiple Holding Registers.vi"("error in (no error)"=w279, "holding register values"=u16[] [95], "starting address"=u16 60 ("write operation starting address"), "Modbus master in"=w280) -> ("error out"=w283:errorcluster, "Modbus master out"=w282:refnum<class "Modbus Master.lvclass">)  [unwired: 6 in]
            n116 = Divide(x=w262) -> (x/y=w268:dbl)  [unwired: 1 in]
            n117 = Multiply(x=w268, y=100.0) -> (x*y=w266:dbl)
            n118 = Multiply(x=w266, y=163.84) -> (x*y=w264:dbl)
            n119 = Build Array(w264) -> (w263:dbl[])
            n120 = call-dynamic "Write Multiple Holding Registers.vi"("error in (no error)"=w283, "holding register values"=w263, "starting address"=u16 704, "Modbus master in"=w282) -> ("error out"=w277:errorcluster, "Modbus master out"=w278:refnum<class "Modbus Master.lvclass">)  [unwired: 6 in]
          }
          frame Enabled {
          }
        }
      }
      frame "Set Velocità" {
        # "0-10000"
        n121 = call-dynamic "Read Holding Registers.vi"("error in (no error)"=w306, "number of holding registers"=u16 1, "starting address"=u16 1710, "Modbus master in"=w307) -> ("error out"=w298:errorcluster, "register values"=w300:u16[], "Modbus master out"=w299:refnum<class "Modbus Master.lvclass">)  [unwired: 5 in]
        n122 = Variant To Data(type=0.0, Variant=w310) -> (data=w290:dbl)  [unwired: 1 in, 1 out]
        n123 = Index Array "n°PAIA POLI"(array=w300) -> (element=w295:u16)  [unwired: 1 in]
        n124 = Divide(x=w290, y=60.0) -> (x/y=w296:dbl)
        n125 = local read "fREQ MAX"() -> (w288:dbl)
        n126 = Multiply(x=w296, y=w295) -> (x*y=w289:dbl)
        n127 = In Range and Coerce(upper limit=w288, x=w289, lower limit=0.0) -> (coerced(x)=w287:dbl)  [unwired: 1 out]
        n128 = Divide(x=w287, y=w288) -> (x/y=w294:dbl)
        n129 = Multiply(x=w294, y=10000.0) -> (x*y=w292:dbl)
        n130 = Build Array(w292) -> (w304:dbl[])
        n131 = call-dynamic "Write Multiple Holding Registers.vi"("error in (no error)"=w298, "holding register values"=w304, "starting address"=u16 2002, "Modbus master in"=w299) -> ("error out"=w311:errorcluster, "Modbus master out"=w312:refnum<class "Modbus Master.lvclass">)  [unwired: 6 in]
        n132 = property class="DigNum (strict)"(reference=w291, "Value"=w290) -> ()  [unwired: 1 in, 2 out]
      }
      frame "Run command" {
        n133 = call-dynamic "Read Holding Registers.vi"("error in (no error)"=w317, "number of holding registers"=u16 1, "starting address"=u16 2000, "Modbus master in"=w316) -> ("error out"=w314:errorcluster, "register values"=w320:u16[], "Modbus master out"=w315:refnum<class "Modbus Master.lvclass">)  [unwired: 5 in]
        n134 = Variant To Data(type=TRUE, Variant=w331) -> (data=w326:bool)  [unwired: 1 in, 1 out]
        n135 = Index Array(array=w320) -> (element=w319:u16)  [unwired: 1 in]
        n136 = Number To Boolean Array(number=w319) -> (Boolean array=w313:bool[])
        n137 = Replace Array Subset(array=w313, new element=w326, index=0) -> (w325:bool[])
        n138 = Boolean Array To Number(Boolean array=w325) -> (number=w324:u32)
        n139 = Build Array(w324) -> (w323:u32[])
        n140 = call-dynamic "Write Multiple Holding Registers.vi"("error in (no error)"=w314, "holding register values"=w323, "starting address"=u16 2000, "Modbus master in"=w315) -> ("error out"=w332:errorcluster, "Modbus master out"=w333:refnum<class "Modbus Master.lvclass">)  [unwired: 6 in]
      }
      frame "Senso rotazione" {
        n141 = disable-structure shown="Disabled" {
          disable-tunnel: w340 -> [w352 _]
          disable-tunnel: w339 -> [w351 _]
          disable-tunnel: [w350 _] -> w338
          disable-tunnel: [w349 _] -> w337
          disable-tunnel: w336 -> [w348 _]
          frame Disabled {
            n142 = Variant To Data(type=TRUE, Variant=w348) -> (data=w345:bool)  [unwired: 1 in, 1 out]
            n143 = call-dynamic "Write Multiple Holding Registers.vi"("error in (no error)"=w351, "holding register values"=u16[] [95], "starting address"=u16 60 ("write operation starting address"), "Modbus master in"=w352) -> ("error out"=w354:errorcluster, "Modbus master out"=w353:refnum<class "Modbus Master.lvclass">)  [unwired: 6 in]
            n144 = Select(t=u16[] [1] ("holding register values"), s=w345, f=u16[] [0] ("holding register values")) -> (s? t:f=w341:u16[])
            n145 = Add(x=76) -> (x+y=w344:i32)  [unwired: 1 in]
            n146 = call-dynamic "Write Multiple Holding Registers.vi"("error in (no error)"=w354, "holding register values"=w341, "starting address"=w344, "Modbus master in"=w353) -> ("error out"=w349:errorcluster, "Modbus master out"=w350:refnum<class "Modbus Master.lvclass">)  [unwired: 6 in]
          }
          frame Enabled {
          }
        }
      }
      frame "Reset allarmi" {
        w359 = u16 2000 ("starting address")
        n147 = call-dynamic "Read Holding Registers.vi"("error in (no error)"=w374, "number of holding registers"=u16 1, "starting address"=w359, "Modbus master in"=w375) -> ("register values"=w372:u16[])  [unwired: 5 in, 2 out]
        n148 = Index Array(array=w372) -> (element=w371:u16)  [unwired: 1 in]
        n149 = Number To Boolean Array(number=w371) -> (Boolean array=w361:bool[])
        n150 = Replace Array Subset(array=w361, new element=TRUE ("new element/subarray"), index=2) -> (w368:bool[])
        n151 = Boolean Array To Number(Boolean array=w368) -> (number=w367:u32)
        n152 = flat-sequence {
          tunnel: w375 -> [w389]
          tunnel: [w388] -> w379
          tunnel: w374 -> [w387]
          tunnel: [w386] -> w378
          tunnel: w366 -> [w385]
          tunnel: w359 -> [w384]
          tunnel: [w384] -> w358
          tunnel: [w392] -> w377
          tunnel: w379 -> [w392]
          tunnel: [w391] -> w376
          tunnel: w378 -> [w391]
          tunnel: w358 -> [w390]
          tunnel: [w390] -> w357
          tunnel: w377 -> [w399]
          tunnel: [w398] -> w383
          tunnel: w376 -> [w397]
          tunnel: [w396] -> w382
          tunnel: w360 -> [w395]
          tunnel: w357 -> [w394]
          frame #0 {
            n153 = call-dynamic "Write Multiple Holding Registers.vi"("error in (no error)"=w387, "holding register values"=w385, "starting address"=w384, "Modbus master in"=w389) -> ("error out"=w386:errorcluster, "Modbus master out"=w388:refnum<class "Modbus Master.lvclass">)  [unwired: 6 in]
          }
          frame #1 {
            n154 = Wait (ms)(milliseconds to wait=u32 500) -> ()  [unwired: 1 out]
          }
          frame #2 {
            n155 = call-dynamic "Write Multiple Holding Registers.vi"("error in (no error)"=w397, "holding register values"=w395, "starting address"=w394, "Modbus master in"=w399) -> ("error out"=w396:errorcluster, "Modbus master out"=w398:refnum<class "Modbus Master.lvclass">)  [unwired: 6 in]
          }
        }
        n156 = Build Array(w367) -> (w366:u32[])
        n157 = Replace Array Subset(array=w361, new element=FALSE ("new element/subarray"), index=2) -> (w364:bool[])
        n158 = Boolean Array To Number(Boolean array=w364) -> (number=w365:u32)
        n159 = Build Array(w365) -> (w360:u32[])
      }
      frame "Close modbus" {
        n160 = flat-sequence {
          tunnel: w404 -> [w405]
          frame #0 {
            n161 = call-dynamic "Close.vi"("Modbus master in"=w405) -> ()  [unwired: 10 in, 1 out]
          }
          frame #1 {
            n162 = Wait (ms)(milliseconds to wait=u32 1500) -> ()  [unwired: 1 out]
          }
        }
        n163 = Enqueue Element(queue=w402, element=cluster{"DATA":variant, "status":string} {"DATA"=variant, "status"="Initialize"}) -> ()  [unwired: 2 in, 3 out]
      }
      frame "Stop" {
        n164 = call-dynamic "Close.vi"("error in (no error)"=w409, "Modbus master in"=w410) -> ()  [unwired: 9 in, 1 out]
      }
      frame "Scelta inverter" {
        n165 = Variant To Data(type=u8 0 ("unit ID"), Variant=w421) -> (data=w413:u8)  [unwired: 1 in, 1 out]
        "id" <- w413
        n166 = Equal?(x=w413, y=u8 3) -> (x = y?=w414:bool)
        n167 = Not Equal To 0?(x=w413) -> (x != 0?=w417:bool)
        n168 = And(x=w417, y=w414) -> (x .and. y?=w415:bool)
        n169 = case shown="True" w415 {
          tunnel: w423 -> [w428 w431]
          tunnel: [w428 w442] -> w422
          tunnel: w413 -> [_ w441]
          tunnel: w419 -> [w426 w439]
          tunnel: w413 -> [_ w434]
          tunnel: w412 -> [_ w433]
          frame False {
            n170 = Flush Queue(queue=w426) -> (queue out=w425:refnum<queue>)  [unwired: 1 in, 2 out]
            n171 = Enqueue Element(queue=w425, element=cluster{"DATA":variant, "status":string} {"DATA"=variant, "status"="IDLE"}) -> ()  [unwired: 2 in, 3 out]
          }
          frame True {
            w437 = u16 0 items=["None", "XON/XOFF", "RTS/CTS", "XON/XOFF & RTS/CTS", "DTR/DSR", "XON/XOFF & DTR/DSR"] ("flow control (None)")
            w436 = u16 0 items=["None", "Odd", "Even"] ("parity (Even)")
            n172 = call-dynamic "Close.vi"("Modbus master in"=w431) -> ("error out"=w430:errorcluster)  [unwired: 10 in]
            n173 = call <vilib>:"Clear Errors.vi"("error in (no error)"=w430) -> ("error out"=w429:errorcluster)  [unwired: 5 in, 1 out]
            n174 = call-poly <vilib>:"Create Master Instance.vi"("flow control (None)"=w437, "serial type"=enum16{"RTU", "ASCII"}."RTU", "parity (Even)"=w436, "unit ID"=w434, "error in (no error)"=w429, "baud rate (9600)"=u32 19200, "VISA resource name"=w433) -> ("serial master instance"=w432:refnum<class "Modbus Master.lvclass">)  [unwired: 3 in, 1 out]
            n175 = property class="Modbus Master"(reference=w432, "Data Access:Unit ID"=w441) -> (reference out=w442:refnum<class "Modbus Master.lvclass">)  [unwired: 1 in, 1 out]
            n176 = Enqueue Element(queue=w439, element=cluster{"DATA":variant, "status":string} {"DATA"=variant, "status"="READ"}) -> ()  [unwired: 2 in, 3 out]
          }
        }
        n177 = property class="Bool (strict)"(reference=w418, "Visible"=w415) -> ()  [unwired: 1 in, 2 out]
      }
      frame "IDLE" {
      }
    }
    "Numeric" <- w54
  }
  n178 = Concatenate Strings(w8, "\\Settings\\Inverter TDE\\opendrive_00_Async_12p2.pct" ("name or relative path")) -> (w6:string)
  n179 = String To Path(string=w6) -> ()  [unwired: 1 out]
  n180 = call-dynamic "Close.vi"("error in (no error)"=w20, "Modbus master in"=w19) -> ()  [unwired: 9 in, 1 out]
